vi "myRIO_BRig_RT__Case_Exp_subState_LC__initTrial__v2.vi"(0 "input_dataCurrent":u16[](array[numeric]), 2 "input_dataLC":u16[](array[numeric]), 6 "input_spout":enum16{"Left", "Right"}(ring), 8 "input_dataTrial":u16[][](array[numeric])) -> (10 "output_dataTrial":u16[][](array[numeric]), 11 "output_LR_Wrong_Laser_l2":bool, 13 "output_LR_Reward_Laser_l2":bool, 14 "output_LR_Reward_Event_l1":bool, 15 "output_LR_Wrong_Event_l1":bool, 16 "output_LR_Reward_Laser_l1":bool, 17 "output_LR_Wrong_Laser_l1":bool, 18 "output_LR_Reward_Event_l2":bool, 19 "output_LR_Wrong_Event_l2":bool)   [LabVIEW 2014]
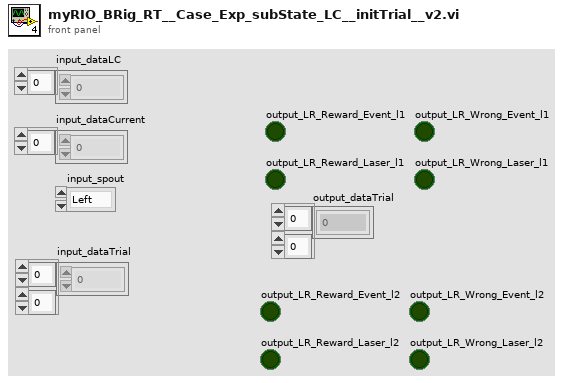
[diagram p1: front panel]
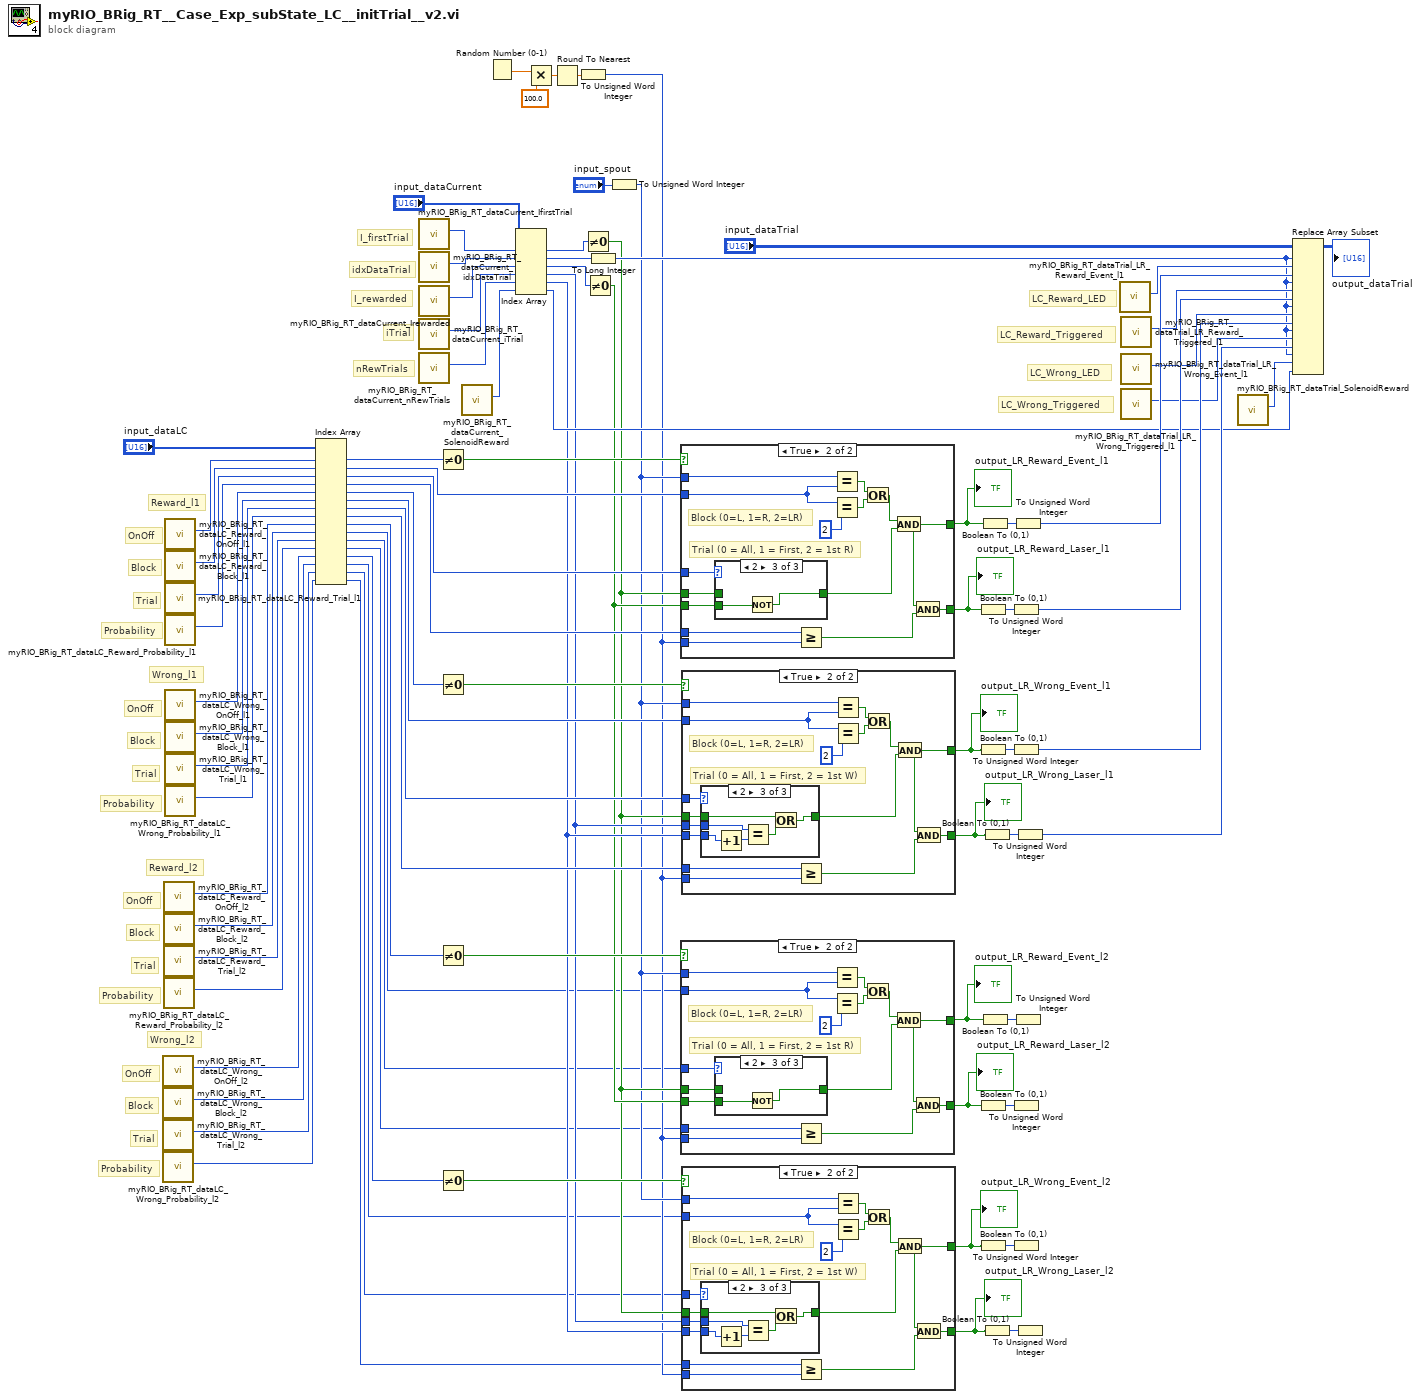
[diagram p0: block diagram]
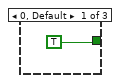
[diagram p3: hidden frame]
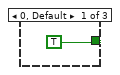
[diagram p6: hidden frame]
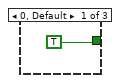
[diagram p9: hidden frame]
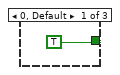
[diagram p12: hidden frame]
diagram:
  # "Probability"
  # "Trial"
  # "Block"
  # "OnOff"
  # "Wrong_l2"
  # "Reward_l2"
  # "Probability"
  # "Trial"
  # "Block"
  # "OnOff"
  # "nRewTrials"
  # "iTrial"
  # "I_rewarded"
  # "LC_Wrong_Triggered"
  # "LC_Wrong_LED"
  # "LC_Reward_Triggered"
  # "LC_Reward_LED"
  # "idxDataTrial"
  # "Probability"
  # "Trial"
  # "Block"
  # "OnOff"
  # "Wrong_l1"
  # "I_firstTrial"
  # "Reward_l1"
  # "Probability"
  # "Trial"
  # "Block"
  # "OnOff"
  n1 = call "myRIO_BRig_RT_dataLC_Wrong_OnOff_l2.vi"() -> ("output_Wrong_OnOff_l2"=w28:i32)  [unwired: 11 in]
  n2 = call "myRIO_BRig_RT_dataLC_Wrong_Block_l2.vi"() -> ("output_Wrong_Block_l2"=w27:i32)  [unwired: 11 in]
  n3 = call "myRIO_BRig_RT_dataLC_Wrong_Trial_l2.vi"() -> ("output_Wrong_Trial_l2"=w26:i32)  [unwired: 11 in]
  n4 = call "myRIO_BRig_RT_dataLC_Wrong_Probability_l2.vi"() -> ("output_Wrong_Probability_l2"=w25:i32)  [unwired: 11 in]
  n5 = call "myRIO_BRig_RT_dataLC_Reward_OnOff_l2.vi"() -> ("output_Reward_OnOff_l2"=w32:i32)  [unwired: 11 in]
  n6 = call "myRIO_BRig_RT_dataLC_Reward_Block_l2.vi"() -> ("output_Reward_Block_l2"=w31:i32)  [unwired: 11 in]
  n7 = call "myRIO_BRig_RT_dataLC_Reward_Trial_l2.vi"() -> ("output_Reward_Trial_l2"=w30:i32)  [unwired: 11 in]
  n8 = call "myRIO_BRig_RT_dataLC_Reward_Probability_l2.vi"() -> ("output_Reward_Probability_l2"=w29:i32)  [unwired: 11 in]
  n9 = call "myRIO_BRig_RT_dataLC_Reward_OnOff_l1.vi"() -> ("output_Reward_OnOff_l1"=w86:i32)  [unwired: 11 in]
  n10 = call "myRIO_BRig_RT_dataLC_Reward_Block_l1.vi"() -> ("output_Reward_Block_l1"=w85:i32)  [unwired: 11 in]
  n11 = call "myRIO_BRig_RT_dataLC_Reward_Trial_l1.vi"() -> ("output_Reward_Trial_l1"=w84:i32)  [unwired: 11 in]
  n12 = call "myRIO_BRig_RT_dataLC_Reward_Probability_l1.vi"() -> ("output_Reward_Probability_l1"=w83:i32)  [unwired: 11 in]
  n13 = call "myRIO_BRig_RT_dataLC_Wrong_OnOff_l1.vi"() -> ("output_Wrong_OnOff_l1"=w71:i32)  [unwired: 11 in]
  n14 = call "myRIO_BRig_RT_dataLC_Wrong_Block_l1.vi"() -> ("output_Wrong_Block_l1"=w72:i32)  [unwired: 11 in]
  n15 = call "myRIO_BRig_RT_dataLC_Wrong_Trial_l1.vi"() -> ("output_Wrong_Trial_l1"=w73:i32)  [unwired: 11 in]
  n16 = call "myRIO_BRig_RT_dataLC_Wrong_Probability_l1.vi"() -> ("output_Wrong_Probability_l1"=w74:i32)  [unwired: 11 in]
  n17 = Index Array(array="input_dataLC", index #1=w86, index #2=w85, index #3=w84, index #4=w83, index #5=w71, index #6=w72, index #7=w73, index #8=w74, index #9=w32, index #10=w31, index #11=w30, index #12=w29, index #13=w28, index #14=w27, index #15=w26, index #16=w25) -> (element #1=w82:u16, element #2=w80:u16, element #3=w79:u16, element #4=w78:u16, element #5=w68:u16, element #6=w67:u16, element #7=w66:u16, element #8=w65:u16, element #9=w8:u16, element #10=w7:u16, element #11=w6:u16, element #12=w5:u16, element #13=w4:u16, element #14=w3:u16, element #15=w2:u16, element #16=w1:u16)
  n18 = call "myRIO_BRig_RT_dataCurrent_IfirstTrial.vi"() -> ("output_I_firstTrial"=w76:i32)  [unwired: 11 in]
  n19 = call "myRIO_BRig_RT_dataCurrent_idxDataTrial.vi"() -> ("output_idxDataTrial"=w64:i32)  [unwired: 11 in]
  n20 = call "myRIO_BRig_RT_dataCurrent_Irewarded.vi"() -> ("output_I_rewarded"=w44:i32)  [unwired: 11 in]
  n21 = call "myRIO_BRig_RT_dataCurrent_iTrial.vi"() -> ("output_iTrial"=w42:i32)  [unwired: 11 in]
  n22 = call "myRIO_BRig_RT_dataCurrent_nRewTrials.vi"() -> ("output_nRewTrials"=w41:i32)  [unwired: 11 in]
  n23 = Not Equal To 0?(x=w82) -> (x != 0?=w81:bool)
  n24 = Not Equal To 0?(x=w68) -> (x != 0?=w69:bool)
  n25 = Not Equal To 0?(x=w8) -> (x != 0?=w24:bool)
  n26 = Not Equal To 0?(x=w4) -> (x != 0?=w23:bool)
  n27 = call "myRIO_BRig_RT_dataCurrent_SolenoidReward.vi"() -> ("output_SolenoidReward"=w40:i32)  [unwired: 11 in]
  n28 = Random Number (0-1)() -> (number: 0 to 1=w33:dbl)
  n29 = Index Array(array="input_dataCurrent", index #1=w76, index #2=w64, index #3=w44, index #4=w42, index #5=w41, index #6=w40) -> (element #1=w75:u16, element #2=w63:u16, element #3=w43:u16, element #4=w13:u16, element #5=w14:u16, element #6=w37:u16)
  n30 = Multiply(x=w33, y=100.0) -> (x*y=w34:dbl)
  n31 = Round To Nearest(number=w34) -> (nearest integer value=w35:dbl)
  n32 = To Unsigned Word Integer(number=w35) -> (unsigned 16bit integer=w9:u16)
  n33 = Not Equal To 0?(x=w75) -> (x != 0?=w11:bool)
  n34 = Not Equal To 0?(x=w43) -> (x != 0?=w12:bool)
  n35 = To Long Integer(number=w63) -> (32bit integer=w39:i32)
  n36 = To Unsigned Word Integer(number="input_spout") -> (unsigned 16bit integer=w10:u16)
  n37 = case shown="True" w81 {
    tunnel: w80 -> [_ w98]
    tunnel: w79 -> [_ w92]
    tunnel: w78 -> [_ w99]
    tunnel: [_ w95] -> w55
    tunnel: [_ w94] -> w59
    tunnel: w10 -> [_ w93]
    tunnel: w12 -> [_ w89]
    tunnel: w11 -> [_ w91]
    tunnel: w9 -> [_ w88]
    frame False {
    }
    frame True {
      # "Block (0=L, 1=R, 2=LR)"
      # "Trial (0 = All, 1 = First, 2 = 1st R)"
      n38 = case shown="2" w92 {
        tunnel: w91 -> [_ w104 _]
        tunnel: [TRUE w104 w105] -> w90
        tunnel: w89 -> [_ _ w106]
        frame 0, Default {
        }
        frame 1 {
        }
        frame 2 {
          n39 = Not(x=w106) -> (.not. x?=w105:bool)
        }
      }
      n40 = Greater Or Equal?(x=w99, y=w88) -> (x >= y?=w97:bool)
      n41 = Equal?(x=w93, y=w98) -> (x = y?=w101:bool)
      n42 = Equal?(x=w98, y=u16 2) -> (x = y?=w100:bool)
      n43 = Or(x=w101, y=w100) -> (x .or. y?=w96:bool)
      n44 = And(x=w96, y=w90) -> (x .and. y?=w94:bool)
      n45 = And(x=w94, y=w97) -> (x .and. y?=w95:bool)
    }
  }
  "output_LR_Reward_Laser_l1" <- w55
  "output_LR_Reward_Event_l1" <- w59
  n46 = case shown="True" w24 {
    tunnel: w7 -> [_ w117]
    tunnel: w6 -> [_ w111]
    tunnel: w5 -> [_ w118]
    tunnel: [_ w114] -> w19
    tunnel: [_ w113] -> w22
    tunnel: w10 -> [_ w112]
    tunnel: w12 -> [_ w108]
    tunnel: w11 -> [_ w110]
    tunnel: w9 -> [_ w107]
    frame False {
    }
    frame True {
      # "Block (0=L, 1=R, 2=LR)"
      # "Trial (0 = All, 1 = First, 2 = 1st R)"
      n47 = case shown="2" w111 {
        tunnel: w110 -> [_ w123 _]
        tunnel: [TRUE w123 w124] -> w109
        tunnel: w108 -> [_ _ w125]
        frame 0, Default {
        }
        frame 1 {
        }
        frame 2 {
          n48 = Not(x=w125) -> (.not. x?=w124:bool)
        }
      }
      n49 = Greater Or Equal?(x=w118, y=w107) -> (x >= y?=w116:bool)
      n50 = Equal?(x=w112, y=w117) -> (x = y?=w120:bool)
      n51 = Equal?(x=w117, y=u16 2) -> (x = y?=w119:bool)
      n52 = Or(x=w120, y=w119) -> (x .or. y?=w115:bool)
      n53 = And(x=w115, y=w109) -> (x .and. y?=w113:bool)
      n54 = And(x=w113, y=w116) -> (x .and. y?=w114:bool)
    }
  }
  "output_LR_Reward_Laser_l2" <- w19
  "output_LR_Reward_Event_l2" <- w22
  n55 = case shown="True" w69 {
    tunnel: w67 -> [_ w137]
    tunnel: w66 -> [_ w131]
    tunnel: w65 -> [_ w138]
    tunnel: [_ w134] -> w46
    tunnel: [_ w133] -> w50
    tunnel: w10 -> [_ w132]
    tunnel: w11 -> [_ w129]
    tunnel: w13 -> [_ w128]
    tunnel: w14 -> [_ w127]
    tunnel: w9 -> [_ w126]
    frame False {
    }
    frame True {
      # "Block (0=L, 1=R, 2=LR)"
      # "Trial (0 = All, 1 = First, 2 = 1st W)"
      n56 = case shown="2" w131 {
        tunnel: [TRUE w143 w148] -> w130
        tunnel: w129 -> [_ w143 w149]
        tunnel: w128 -> [_ _ w145]
        tunnel: w127 -> [_ _ w147]
        frame 0, Default {
        }
        frame 1 {
        }
        frame 2 {
          n57 = Increment(x=w147) -> (x+1=w146:u16)
          n58 = Equal?(x=w145, y=w146) -> (x = y?=w144:bool)
          n59 = Or(x=w149, y=w144) -> (x .or. y?=w148:bool)
        }
      }
      n60 = Greater Or Equal?(x=w138, y=w126) -> (x >= y?=w136:bool)
      n61 = Equal?(x=w132, y=w137) -> (x = y?=w140:bool)
      n62 = Equal?(x=w137, y=u16 2) -> (x = y?=w139:bool)
      n63 = Or(x=w140, y=w139) -> (x .or. y?=w135:bool)
      n64 = And(x=w135, y=w130) -> (x .and. y?=w133:bool)
      n65 = And(x=w133, y=w136) -> (x .and. y?=w134:bool)
    }
  }
  "output_LR_Wrong_Laser_l1" <- w46
  "output_LR_Wrong_Event_l1" <- w50
  n66 = case shown="True" w23 {
    tunnel: w3 -> [_ w161]
    tunnel: w2 -> [_ w155]
    tunnel: w1 -> [_ w162]
    tunnel: [_ w158] -> w15
    tunnel: [_ w157] -> w17
    tunnel: w10 -> [_ w156]
    tunnel: w11 -> [_ w153]
    tunnel: w13 -> [_ w152]
    tunnel: w14 -> [_ w151]
    tunnel: w9 -> [_ w150]
    frame False {
    }
    frame True {
      # "Block (0=L, 1=R, 2=LR)"
      # "Trial (0 = All, 1 = First, 2 = 1st W)"
      n67 = case shown="2" w155 {
        tunnel: [TRUE w167 w172] -> w154
        tunnel: w153 -> [_ w167 w173]
        tunnel: w152 -> [_ _ w169]
        tunnel: w151 -> [_ _ w171]
        frame 0, Default {
        }
        frame 1 {
        }
        frame 2 {
          n68 = Increment(x=w171) -> (x+1=w170:u16)
          n69 = Equal?(x=w169, y=w170) -> (x = y?=w168:bool)
          n70 = Or(x=w173, y=w168) -> (x .or. y?=w172:bool)
        }
      }
      n71 = Greater Or Equal?(x=w162, y=w150) -> (x >= y?=w160:bool)
      n72 = Equal?(x=w156, y=w161) -> (x = y?=w164:bool)
      n73 = Equal?(x=w161, y=u16 2) -> (x = y?=w163:bool)
      n74 = Or(x=w164, y=w163) -> (x .or. y?=w159:bool)
      n75 = And(x=w159, y=w154) -> (x .and. y?=w157:bool)
      n76 = And(x=w157, y=w160) -> (x .and. y?=w158:bool)
    }
  }
  "output_LR_Wrong_Laser_l2" <- w15
  "output_LR_Wrong_Event_l2" <- w17
  n77 = Boolean To (0,1)(Boolean=w55) -> (0, 1=w56:i16)
  n78 = Boolean To (0,1)(Boolean=w50) -> (0, 1=w51:i16)
  n79 = Boolean To (0,1)(Boolean=w19) -> (0, 1=w20:i16)
  n80 = Boolean To (0,1)(Boolean=w17) -> (0, 1=w18:i16)
  n81 = Boolean To (0,1)(Boolean=w59) -> (0, 1=w58:i16)
  n82 = Boolean To (0,1)(Boolean=w22) -> (0, 1=w21:i16)
  n83 = Boolean To (0,1)(Boolean=w46) -> (0, 1=w47:i16)
  n84 = Boolean To (0,1)(Boolean=w15) -> (0, 1=w16:i16)
  n85 = To Unsigned Word Integer(number=w56) -> (unsigned 16bit integer=w53:u16)
  n86 = To Unsigned Word Integer(number=w51) -> (unsigned 16bit integer=w49:u16)
  n87 = To Unsigned Word Integer(number=w20) -> ()  [unwired: 1 out]
  n88 = To Unsigned Word Integer(number=w18) -> ()  [unwired: 1 out]
  n89 = To Unsigned Word Integer(number=w58) -> (unsigned 16bit integer=w57:u16)
  n90 = To Unsigned Word Integer(number=w21) -> ()  [unwired: 1 out]
  n91 = To Unsigned Word Integer(number=w47) -> (unsigned 16bit integer=w45:u16)
  n92 = To Unsigned Word Integer(number=w16) -> ()  [unwired: 1 out]
  n93 = call "myRIO_BRig_RT_dataTrial_LR_Reward_Event_l1.vi"() -> ("output_LR_Reward_Event_l1"=w60:i32)  [unwired: 11 in]
  n94 = call "myRIO_BRig_RT_dataTrial_LR_Reward_Triggered_l1.vi"() -> ("output_LR_Reward_Triggered_l1"=w54:i32)  [unwired: 11 in]
  n95 = call "myRIO_BRig_RT_dataTrial_LR_Wrong_Event_l1.vi"() -> ("output_LR_Wrong_Event_l1"=w52:i32)  [unwired: 11 in]
  n96 = call "myRIO_BRig_RT_dataTrial_LR_Wrong_Triggered_l1.vi"() -> ("output_LR_Wrong_Triggered_l1"=w48:i32)  [unwired: 11 in]
  n97 = call "myRIO_BRig_RT_dataTrial_SolenoidReward.vi"() -> ("output_SolenoidReward"=w38:i32)  [unwired: 11 in]
  n98 = Replace Array Subset(array="input_dataTrial", new element #1=w57, index (row) #1=w39, index (col) #1=w60, new element #2=w53, index (row) #2=w39, index (col) #2=w54, new element #3=w49, index (row) #3=w39, index (col) #3=w52, new element #4=w45, index (row) #4=w39, index (col) #4=w48, new element #5=w37, index (row) #5=w39, index (col) #5=w38) -> (→"output_dataTrial":u16[][])
